vi "Send Global Chat.vi"(8 "error in (no error)":errorcluster, 10 "Message":string, 11 "Server in":refnum<class "Server.lvclass">) -> (0 "error out":errorcluster, 3 "Server out":refnum<class "Server.lvclass">)   [LabVIEW 2020, in "Server.lvlib" / "Server.lvclass"]
uses:
  Server.lvclass
  Server.lvclass/Server.ctl
  Chat Window Model/Chat Window Model Messages/New Message Msg/New Message Msg.lvclass/New Message Msg.ctl
  <vilib>/ActorFramework/Message Enqueuer/Message Enqueuer.lvclass/Message Enqueuer.ctl
  <vilib>/ActorFramework/Message Enqueuer/Enqueue.vi
  Chat Window Model/Chat Window Model Messages/New Message Msg/New Message Msg.lvclass
  C:/Program Files/National Instruments/LabVIEW 2020/vi.lib/ActorFramework/Message/Message.lvclass
  <vilib>/ActorFramework/Message Priority Queue/Priority Enqueue.vi
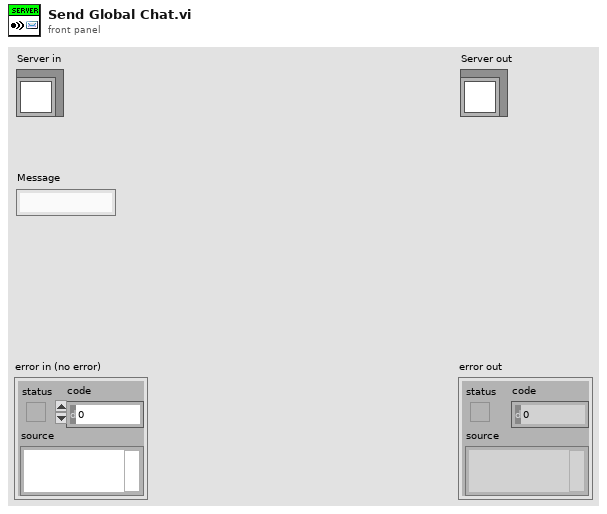
[diagram p1: front panel]
types:
  T1 = map{string, cluster{"Enqueuer":refnum<class "Message Enqueuer.lvclass">, "Status":string}}
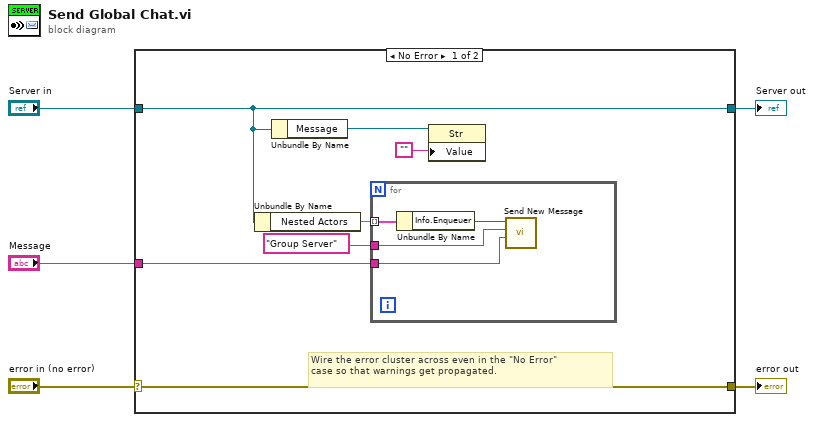
[diagram p0: block diagram]
diagram:
  n1 = case shown="No Error" "error in (no error)" {
    selector: "error in (no error)" -> [w12 w18]
    tunnel: [w12 w18] -> w4
    tunnel: [w8 w17] -> w2
    tunnel: "Server in" -> [w8 w17]
    tunnel: "Message" -> [w11 _]
    frame No Error {
      # "Wire the error cluster across even in the \"No Error\"\ncase so that warnings get propagated."
      n2 = Unbundle By Name(w8) -> ("Nested Actors"=w9:T1)
      n3 = Unbundle By Name(w8) -> ("Message"=w7:refnum<vi>)
      n4 = for {
        tunnel: w9 -> [w16] mode=indexing
        tunnel: w11 -> [w15]
        tunnel: "Group Server" -> [w14]
        n5 = Unbundle By Name(w16) -> ("Info.Enqueuer"=w13:refnum<class "Message Enqueuer.lvclass">)
        n6 = call "Send New Message.vi"("New Message"=w15, "From"=w14, "Message Enqueuer"=w13) -> ()  [unwired: 7 in, 2 out]
      }
      n7 = property class="Str"(reference=w7, "Value"="") -> ()  [unwired: 1 in, 2 out]
    }
    frame Error {
    }
  }
  "error out" <- w4
  "Server out" <- w2
